vi "Format 5.3.vi"(5 "Force Safe Mode (F)":bool, 6 "Timeout (300,000 ms)":u32=300000, 7 "Restart After Format (T)":bool=TRUE, 8 "error in (no error)":errorcluster, 9 "Network Settings (reset all adapters)":T1 items=["reset all network adapters", "preserve primary, reset others", "preserve all network adapters"], 10 "File System":T2 items=["Default"=0, "FAT"=1, "Reliance"=2, "UBIFS"=16384, "Ext4"=32768], 11 "Session in":refnum<k21>) -> (0 "error out":errorcluster, 3 "Session out":refnum<k21>)   [LabVIEW 2017, in "nisyscfg.lvlib"]
doc: "Erases all data from the primary hard drive of a system. If the system is not in user-directed safe mode, and the target's boot flow requires the target to be in safe mode prior to executing the format operation, then this VI will return an error unless <B>force safe mode</B> is TRUE. Refer to the the definition of safe mode to understand the differences between safe mode for different target boot flows."
uses:
  <vilib>/nisyscfg/nisyscfg.lvlib
  <vilib>/nisyscfg/File System.ctl
  <vilib>/nisyscfg/Network Settings Format.ctl
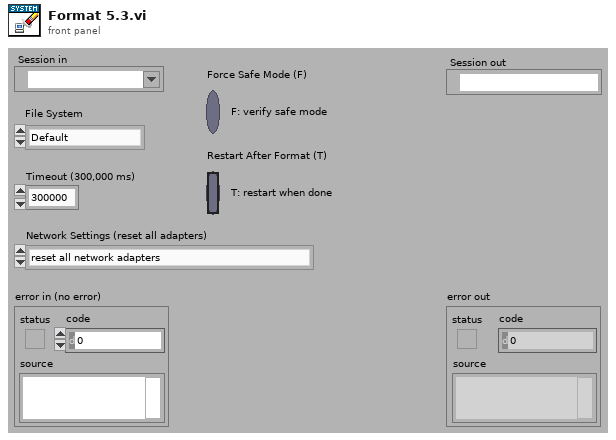
[diagram p1: front panel]
types:
  T1 = typedef "nisyscfg.lvlib/Network Settings Format.ctl" = u32
  T2 = typedef "nisyscfg.lvlib/File System.ctl" = i32
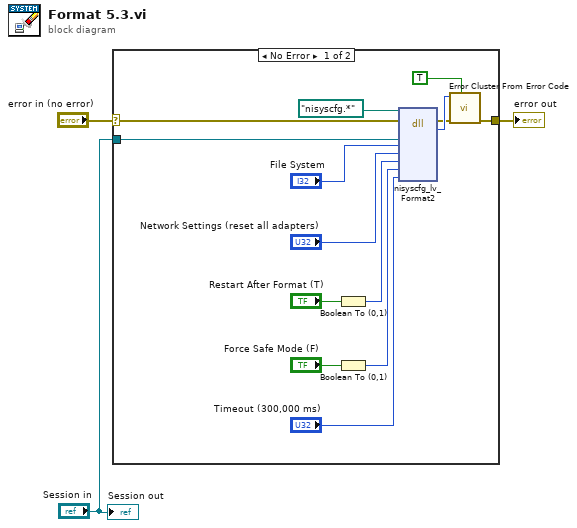
[diagram p0: block diagram]
diagram:
  n1 = case shown="No Error" "error in (no error)" {
    selector: "error in (no error)" -> [w11 w18]
    tunnel: "Session in" -> [w10 _]
    tunnel: [w9 w18] -> w3
    frame No Error {
      n2 = Boolean To (0,1)(Boolean="Restart After Format (T)") -> (0, 1=w8:i16)
      n3 = Boolean To (0,1)(Boolean="Force Safe Mode (F)") -> (0, 1=w5:i16)
      n4 = dll-call lib="nisyscfg.*" fn="nisyscfg_lv_Format2" label="Format"(path in=path "nisyscfg.*", error in=w11, "system"=w10, "fileSystem"="File System", "networkSettings"="Network Settings (reset all adapters)", "restartAfterFormat"=w8, "forceSafeMode"=w5, "timeout"="Timeout (300,000 ms)") -> (error out=w16:errorcluster, "result"=w17:i32)  [unwired: 7 in, 1 out]
      n5 = call <vilib>:"Error Cluster From Error Code.vi"("show call chain? (False)"=TRUE, "error in (no error)"=w16, "error code (0)"=w17) -> ("error out"=w9:errorcluster)  [unwired: 6 in]
    }
    frame Error {
    }
  }
  "error out" <- w3
  "Session out" <- "Session in"
